vi "SParam custom dialog.vi"(11 "Message":string) -> ()   [LabVIEW 2023]
panel:
  out "Message 2":string
  in  "OK Button":bool
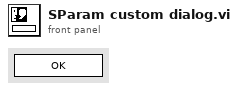
[diagram p1: front panel]
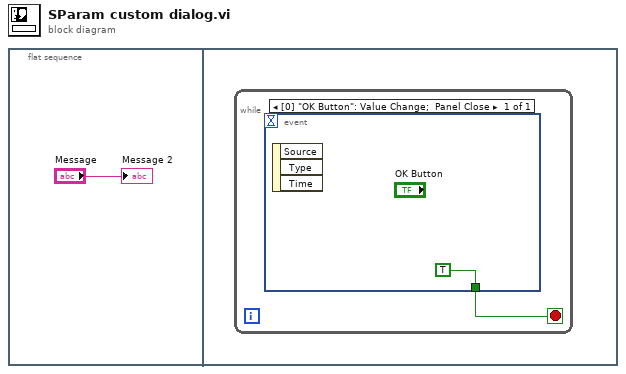
[diagram p0: block diagram]
diagram:
  n1 = flat-sequence {
    frame #0 {
      "Message 2" <- "Message"
    }
    frame #1 {
      n2 = while {
        stop <- w2 stop-if-true
        n3 = event shown="[0] \"OK Button\": Value Change;  Panel Close" {
          selector: _ -> [_]
          dyn-events: _ -> [_]
          timeout: _ -> [_]
          tunnel: [TRUE] -> w2
          event "OK Button": Value Change; Panel Close {
            n4 = event-data() -> ()  [unwired: 1 in, 3 out]
          }
        }
      }
    }
  }
